vi "CarControl.vi"() -> ()   [LabVIEW 2012]
uses:
  <vilib>/RTI DDS Toolkit for LabVIEW/Library/LVDDS_library.lvlib
  <vilib>/RTI DDS Toolkit for LabVIEW/VIs/Read_Num.vi
  <vilib>/RTI DDS Toolkit for LabVIEW/VIs/Write_Num.vi
  <vilib>/RTI DDS Toolkit for LabVIEW/VIs/SimpleCreateReader_NumDbl.vi
  <vilib>/RTI DDS Toolkit for LabVIEW/VIs/SimpleCreateWriter_NumDbl.vi
panel:
  in  "stop":bool
  in  "DomainId":u32
  in  "Brake":dbl(slide) scale=0.0..100.0
  in  "Gas":dbl(slide) scale=0.0..100.0
  out "Distance":dbl
  out "Speed":dbl(knob) scale=0.0..200.0
  # "This pane can modify the values of Gas & Brake.\nAlso, it is receiving the corresponding Speed and \nDistance the car should have."
  # "The DomainId should be set\nbefore run the application"
  # "Sent data"
  # "Received data"
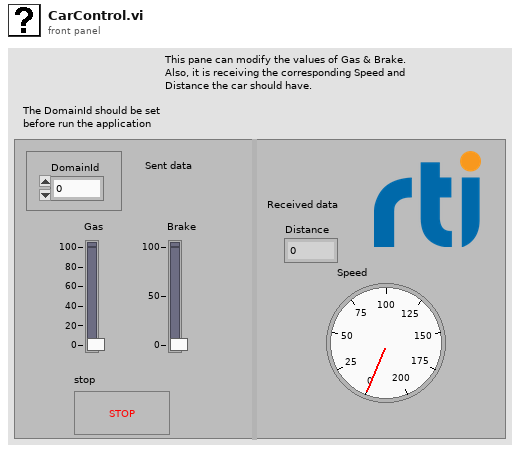
[diagram p1: front panel]
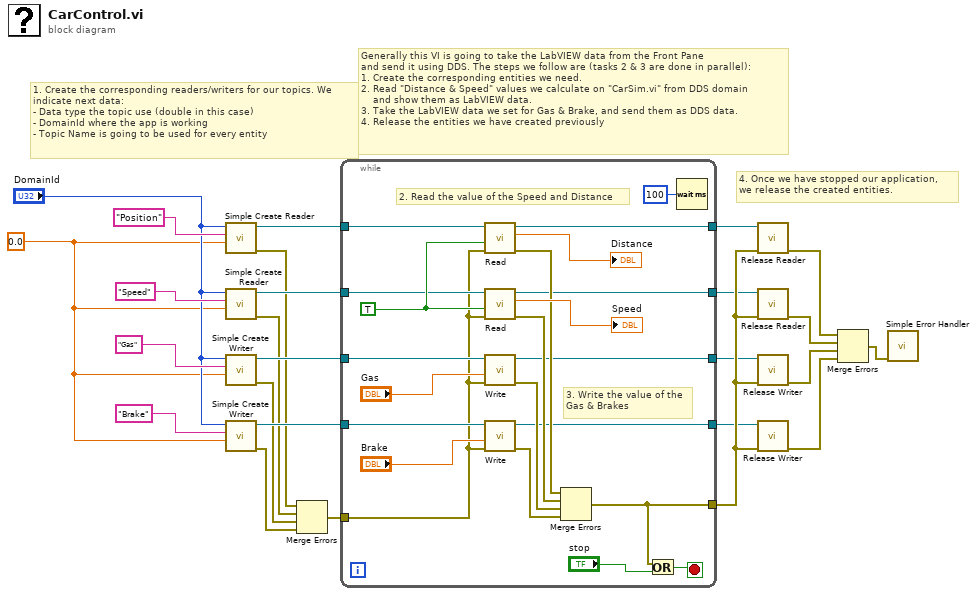
[diagram p0: block diagram]
diagram:
  w16 = 0.0
  # "4. Once we have stopped our application,\nwe release the created entities."
  # "1. Create the corresponding readers/writers for our topics. We\nindicate next data:\n- Data type the topic use (double in this case)\n- DomainId where the app is working\n- Topic Name is going to be used for every entity"
  # "Generally this VI is going to take the LabVIEW data from the Front Pane\nand send it using DDS. The steps we follow are (tasks 2 & 3 are done in parallel):\n1. Create the corresponding entities we need.\n2. Read \"Distance & Speed\" values we calculate on \"CarSim.vi\" from DDS domain\n    and show them as LabVIEW data.\n3. Take the LabVIEW data we set for Gas & Brake, and send them as DDS data.\n4. Release the entities we have created previously"
  n1 = call-poly <vilib>:"Simple Create Reader.vi"("data type"=w16, "topic name"="Position", "domain id"="DomainId") -> ("error out"=w15:errorcluster, "dds read object ref"=w24:refnum<k1>)  [unwired: 7 in]
  n2 = call-poly <vilib>:"Simple Create Reader.vi"("data type"=w16, "topic name"="Speed", "domain id"="DomainId") -> ("error out"=w14:errorcluster, "dds read object ref"=w23:refnum<k1>)  [unwired: 7 in]
  n3 = call-poly <vilib>:"Simple Create Writer.vi"("data type"=w16, "topic name"="Gas", "domain id"="DomainId") -> ("error out"=w13:errorcluster, "dds writer object ref"=w21:refnum<k1>)  [unwired: 7 in]
  n4 = call-poly <vilib>:"Simple Create Writer.vi"("data type"=w16, "topic name"="Brake", "domain id"="DomainId") -> ("error out"=w12:errorcluster, "dds writer object ref"=w19:refnum<k1>)  [unwired: 7 in]
  n5 = Merge Errors(w15, w14, w13, w12) -> (w11:errorcluster)
  n6 = while {
    tunnel: w19 -> [w42]
    tunnel: w21 -> [w41]
    tunnel: w23 -> [w40]
    tunnel: w24 -> [w39]
    tunnel: w11 -> [w38]
    tunnel: [w33] -> w9
    tunnel: [w32] -> w8
    tunnel: [w31] -> w7
    tunnel: [w30] -> w6
    tunnel: [w27] -> w10
    stop <- w29 stop-if-true
    w43 = TRUE
    # "3. Write the value of the\nGas & Brakes"
    # "2. Read the value of the Speed and Distance"
    n7 = call-poly <vilib>:"Read.vi"("error in (no error)"=w38, "only_new_samples"=w43, "dds read object ref in"=w39) -> ("error out"=w37:errorcluster, "data"=→"Distance":dbl, "dds read object ref out"=w33:refnum<k1>)  [unwired: 5 in, 1 out]
    n8 = call-poly <vilib>:"Read.vi"("error in (no error)"=w38, "only_new_samples"=w43, "dds read object ref in"=w40) -> ("error out"=w36:errorcluster, "data"=→"Speed":dbl, "dds read object ref out"=w32:refnum<k1>)  [unwired: 5 in, 1 out]
    n9 = call-poly <vilib>:"Write.vi"("error in"=w38, "data"="Gas", "dds write object ref in"=w41) -> ("error out"=w35:errorcluster, "dds write object ref out"=w31:refnum<k1>)  [unwired: 7 in]
    n10 = call-poly <vilib>:"Write.vi"("error in"=w38, "data"="Brake", "dds write object ref in"=w42) -> ("error out"=w34:errorcluster, "dds write object ref out"=w30:refnum<k1>)  [unwired: 7 in]
    n11 = Merge Errors(w37, w36, w35, w34) -> (w27:errorcluster)
    n12 = Or(x=w27, y="stop") -> (x .or. y?=w29:bool)
    n13 = Wait (ms)(milliseconds to wait=u32 100) -> ()  [unwired: 1 out]
  }
  n14 = call <vilib>:"Release Reader.vi"("error in"=w10, "dds read object ref in"=w9) -> ("error out"=w5:errorcluster)  [unwired: 9 in]
  n15 = call <vilib>:"Release Reader.vi"("error in"=w10, "dds read object ref in"=w8) -> ("error out"=w4:errorcluster)  [unwired: 9 in]
  n16 = call <vilib>:"Release Writer.vi"("error in"=w10, "dds write object ref"=w7) -> ("error out"=w3:errorcluster)  [unwired: 9 in]
  n17 = call <vilib>:"Release Writer.vi"("error in"=w10, "dds write object ref"=w6) -> ("error out"=w2:errorcluster)  [unwired: 9 in]
  n18 = Merge Errors(w5, w4, w3, w2) -> (w1:errorcluster)
  n19 = call <vilib>:"Simple Error Handler.vi"("error in (no error)"=w1) -> ()  [unwired: 4 in, 5 out]
